vi "host_set_size.vi"(8 "error in (no error)":errorcluster, 9 "fast":i32=256 min=1, 10 "slow":i32=256 min=1, 11 "page":i32=2 min=1) -> (0 "error out":errorcluster)   [LabVIEW 2021]
doc: "Allocate a 4D array for the scan. A reference for the allocated array is stored as \"data reference\" in host_global_var.vi. \"page\", \"slow\", \"fast\" specify the size of the array."
uses:
  core/host_global_vars.vi
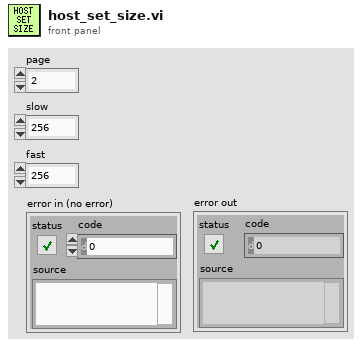
[diagram p1: front panel]
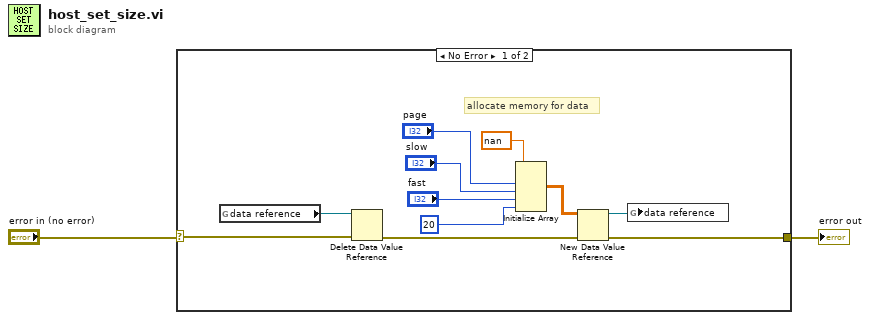
[diagram p0: block diagram]
diagram:
  n1 = case shown="No Error" "error in (no error)" {
    selector: "error in (no error)" -> [w4 w14]
    tunnel: [w3 w14] -> w1
    frame No Error {
      # "allocate memory for data"
      n2 = global read "host_global_vars.vi" "data reference"() -> (w6:refnum<data-value>)
      n3 = Delete Data Value Reference(data value reference=w6, error in=w4) -> (error out=w7:errorcluster)  [unwired: 1 out]
      n4 = Initialize Array(sgl nan, "page", "slow", "fast", 20 ("dimension size")) -> (w13:sgl[][][][])
      n5 = New Data Value Reference(data value=w13, error in=w7) -> (data value reference=w11:refnum<data-value>, error out=w3:errorcluster)
      n6 = global write "host_global_vars.vi" "data reference"(w11) -> ()
    }
    frame Error {
    }
  }
  "error out" <- w1
